vi "lvasketch.vi"() -> ()   [LabVIEW 2021]
doc: "This VI looks very similar to an Etch - a - Sketch. It uses the picture control toolkit to create an image and add points to update the picture with the press of a keyboard button. You may have to 'skake' it a few times."
panel:
  out "Numeric 2":i16
  out "Numeric":i16
  in  "Right":bool
  in  "Left":bool
  in  "Down":bool
  in  "Up":bool
  in  "stop":bool
  in  "Boolean":bool
  in  "PEN COLOR":u32(colorbox)
  out "LABVIEW - a - SKETCH":picture
  out "LEFT - RIGHT":i16(knob) min=0 step=1 scale=0.0..400.0
  out "UP - DOWN":i16(knob) min=0 max=400 step=1 scale=0.0..400.0
  # "F1"
  # "F2"
  # "F7"
  # "F8"
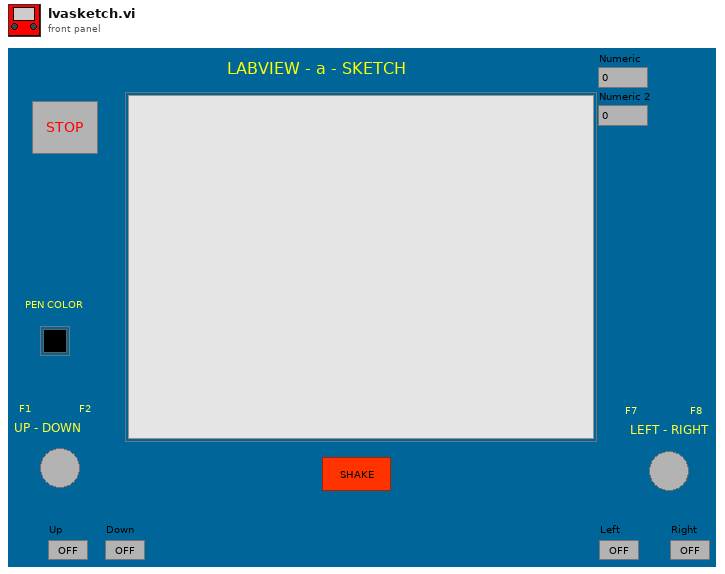
[diagram p1: front panel]
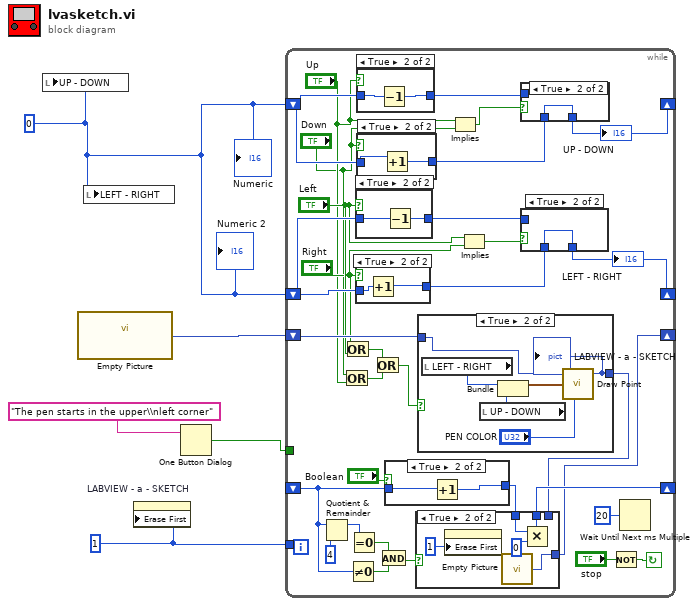
[diagram p0: block diagram]
diagram:
  w5 = u8 1 ("Write Attribute")
  w3 = i16 0
  n1 = local write "UP - DOWN"(w3) -> ()
  n2 = call "Empty Picture"() -> ("empty picture"=w4:picture)
  n3 = local write "LEFT - RIGHT"(w3) -> ()
  n4 = property on="LABVIEW - a - SKETCH" class="Pict"("Erase First"=w5) -> ()  [unwired: 2 in, 2 out]
  n5 = One Button Dialog(message="The pen starts in the upper\\nleft corner") -> (true=w1:bool)  [unwired: 1 in]
  n6 = while {
    tunnel: w1 -> [_]
    shift-left: w3 -> [w19]
    shift-right: [w7] -> _
    shift-left: w3 -> [w18]
    shift-right: [w15] -> _
    tunnel: w5 -> [_]
    shift-left: _ -> [w28]
    shift-right: [w22] -> _
    shift-left: w4 -> [w32]
    shift-right: [w20] -> _
    stop <- w36 continue-if-true
    n7 = Quotient & Remainder(x=w28, y=4) -> (x-y*floor(x/y)=w29:i32)  [unwired: 1 out]
    n8 = Or(x="Down", y="Up") -> (x .or. y?=w35:bool)
    n9 = Or(x="Right", y="Left") -> (x .or. y?=w34:bool)
    n10 = Not Equal To 0?(x=w28) -> (x != 0?=w27:bool)
    n11 = Equal To 0?(x=w29) -> (x = 0?=w26:bool)
    n12 = case shown="True" "Left" {
      tunnel: w18 -> [w62 w64]
      tunnel: [w62 w63] -> w17
      frame False {
      }
      frame True {
        n13 = Decrement(x=w64) -> (x-1=w63:i16)
      }
    }
    n14 = case shown="True" "Right" {
      tunnel: w18 -> [w59 w61]
      tunnel: [w59 w60] -> w16
      frame False {
      }
      frame True {
        n15 = Increment(x=w61) -> (x+1=w60:i16)
      }
    }
    n16 = case shown="True" "Up" {
      tunnel: w19 -> [w68 w70]
      tunnel: [w68 w69] -> w11
      frame False {
      }
      frame True {
        n17 = Decrement(x=w70) -> (x-1=w69:i16)
      }
    }
    n18 = case shown="True" "Down" {
      tunnel: w19 -> [w65 w67]
      tunnel: [w65 w66] -> w8
      frame False {
      }
      frame True {
        n19 = Increment(x=w67) -> (x+1=w66:i16)
      }
    }
    n20 = Or(x=w34, y=w35) -> (x .or. y?=w33:bool)
    n21 = And(x=w26, y=w27) -> (x .and. y?=w25:bool)
    n22 = case shown="True" "Boolean" {
      tunnel: w28 -> [w42 w44]
      tunnel: [w42 w43] -> w23
      frame False {
      }
      frame True {
        n23 = Increment(x=w44) -> (x+1=w43:i32)
      }
    }
    n24 = case shown="True" w33 {
      tunnel: w32 -> [w52 w57]
      tunnel: [w52 w56] -> w21
      frame False {
      }
      frame True {
        n25 = local read "LEFT - RIGHT"() -> (w55:i16)
        n26 = local read "UP - DOWN"() -> (w54:i16)
        n27 = Bundle("LEFT - RIGHT"=w55, "UP - DOWN"=w54) -> (w53:cluster{"LEFT - RIGHT":i16, "UP - DOWN":i16})  [unwired: 1 in]
        n28 = call <vilib>:"Draw Point.vi"("picture"=w57, "point(x,y)"=w53, "color(black)"="PEN COLOR") -> ("new picture"=w56:picture)  [unwired: 6 in]
        "LABVIEW - a - SKETCH" <- w56
      }
    }
    n29 = case shown="True" w25 {
      tunnel: w23 -> [w46 w50]
      tunnel: [w46 w49] -> w22
      tunnel: w21 -> [w45 _]
      tunnel: [w45 w48] -> w20
      frame False {
      }
      frame True {
        n30 = property on="LABVIEW - a - SKETCH" class="Pict"("Erase First"=u8 1 ("Write Attribute")) -> ()  [unwired: 2 in, 2 out]
        n31 = call "Empty Picture"() -> ("empty picture"=w48:picture)
        n32 = Multiply(x=w50, y=0) -> (x*y=w49:i32)
      }
    }
    n33 = Implies(1:"Down", 2:"Up") -> (0:w6:bool)
    n34 = Implies(1:"Right", 2:"Left") -> (0:w12:bool)
    n35 = case shown="True" w6 {
      tunnel: w11 -> [w38 _]
      tunnel: w8 -> [_ w39]
      tunnel: [w38 w39] -> w7
      frame False {
      }
      frame True {
      }
    }
    "UP - DOWN" <- w7
    n36 = case shown="True" w12 {
      tunnel: w17 -> [w40 _]
      tunnel: w16 -> [_ w41]
      tunnel: [w40 w41] -> w15
      frame False {
      }
      frame True {
      }
    }
    "LEFT - RIGHT" <- w15
    n37 = Not(x="stop") -> (.not. x?=w36:bool)
    n38 = Wait Until Next ms Multiple(millisecond multiple=u32 20) -> ()  [unwired: 1 out]
  }
  "Numeric" <- w3
  "Numeric 2" <- w3
